vi "Configuration - Read First Analog In Configuration.vi"(8 "error in":errorcluster, 11 "Carrier Configuration":T1={"Name"="Default Settings", "IP"="192.168.0.84", "Control Port"=4220, "Timeout (ms)"=2000, "Continuous Capture Port (Multiplexed)"=4210, "Start HIL Shot Port"=53999, "AWG Upload Port (Multiplexed)"=54201, "Download Captured Data Port (Multiplexed)"=53000, "Module Slots"=2, "Module Configurations"=[{"Name"="ACQ 425 ELF", "Position"="192.168.0.84", "Module Type"=enum."Analog In Module", "Control Port"=4221, "Timeout (ms)"=2000, "Channels"=16}, {"Name"="AO 424 ELF", "Position"="192.168.0.84", "Module Type"=enum."Analog Out Module", "Control Port"=4222, "Timeout (ms)"=2000, "Channels"=16}]}) -> (0 "error out":errorcluster, 1 "Timeout (ms)":i32, 2 "Analog In Control Port":i32, 3 "Carrier Control Port":i32, 5 "AI - Module Configuration":T2)   [LabVIEW 2017, in "Communications Library.lvlib"]
uses:
  Communications Library.lvlib
  Typedefs/DTACQ Module Configuration--Cluster.ctl
  Typedefs/DTACQ Device Type--Enum.ctl
  Typedefs/DTACQ Module Carrier Configuration--Cluster.ctl
  <vilib>/Utility/error.llb/Error Cluster From Error Code.vi
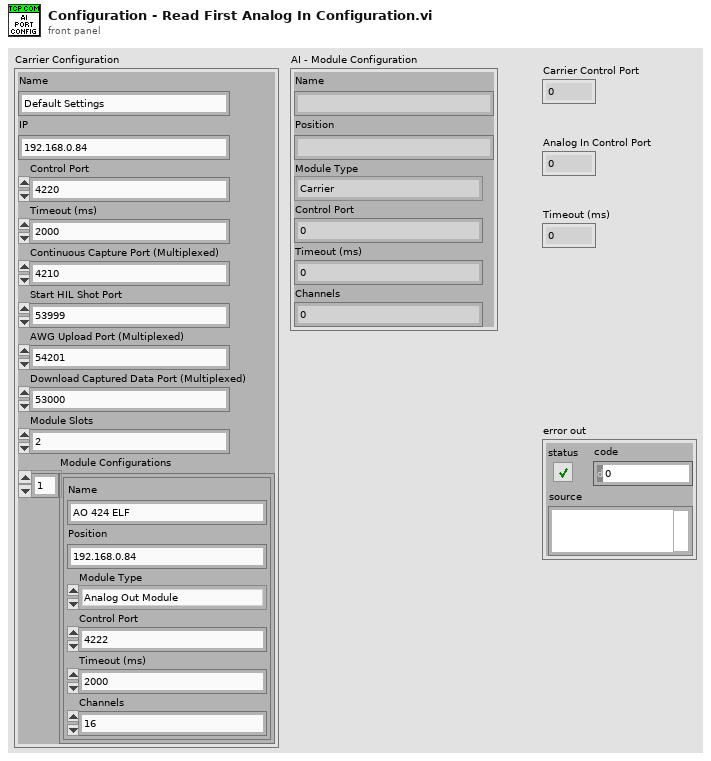
[diagram p1: front panel]
types:
  T1 = typedef "Communications Library.lvlib/DTACQ Module Carrier Configuration--Cluster.ctl" = cluster{"Name":string, "IP":string, "Control Port":i32, "Timeout (ms)":i32, "Continuous Capture Port (Multiplexed)":i32, "Start HIL Shot Port":i32, "AWG Upload Port (Multiplexed)":i32, "Download Captured Data Port (Multiplexed)":i32, "Module Slots":i32, "Module Configurations":T2[]}
  T2 = typedef "Communications Library.lvlib/DTACQ Module Configuration--Cluster.ctl" = cluster{"Name":string, "Position":string, "Module Type":T3, "Control Port":i32, "Timeout (ms)":i32, "Channels":i32}
  T3 = typedef "Communications Library.lvlib/DTACQ Device Type--Enum.ctl" = enum16{"Carrier", "Analog In Module", "Analog Out Module", "Generic Module"}
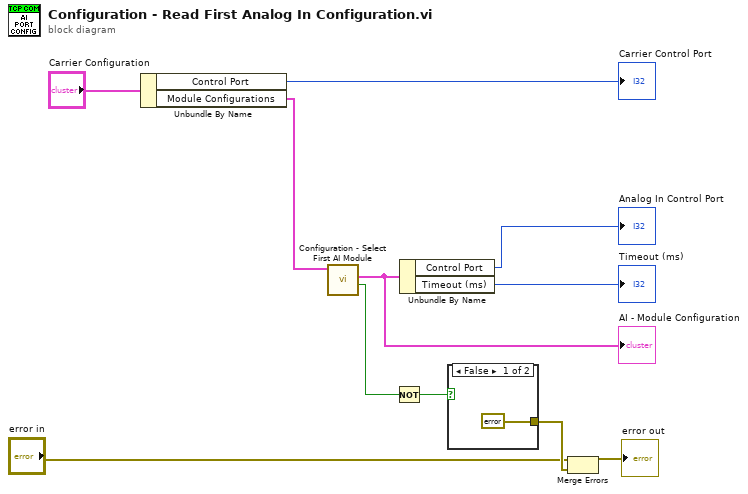
[diagram p0: block diagram]
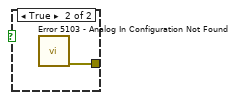
[diagram p2: hidden frame]
diagram:
  n1 = Unbundle By Name("Carrier Configuration") -> ("Control Port"=→"Carrier Control Port":i32, "Module Configurations"=w11:T2[])
  n2 = call "Configuration - Select First AI Module.vi"("Module Configurations"=w11) -> ("AI Found"=w5:bool, "Module Configuration"=w2:T2)  [unwired: 9 in]
  "AI - Module Configuration" <- w2
  n3 = Not(x=w5) -> (.not. x?=w6:bool)
  n4 = Unbundle By Name(w2) -> ("Control Port"=→"Analog In Control Port":i32, "Timeout (ms)"=→"Timeout (ms)":i32)
  n5 = case shown="False" w6 {
    tunnel: [errorcluster {"status"=FALSE, "code"=0, "source"=""} ("error out") w13] -> w9
    frame False {
    }
    frame True {
      n6 = call "Error 5103 - Analog In Configuration Not Found.vi"() -> ("error out"=w13:errorcluster)  [unwired: 11 in]
    }
  }
  n7 = Merge Errors("error in", w9) -> (→"error out":errorcluster)
